vi "stdin.write.vi"(8 "error in (no error)":errorcluster, 10 "stdin":string, 11 "dotnet_system_exec in":refnum<class "dotnet_system_exec.lvclass">) -> (0 "error out":errorcluster, 3 "dotnet_system_exec out":refnum<class "dotnet_system_exec.lvclass">)   [LabVIEW 2015, in "dotnet_system_exec.lvclass"]
doc: "Sends a line to the .NET process via stdin. This vi accepts multiline inputs in case multiple lines want to be sent at once."
uses:
  dotnet_system_exec.lvclass
  dotnet_system_exec.lvclass/dotnet_system_exec.ctl
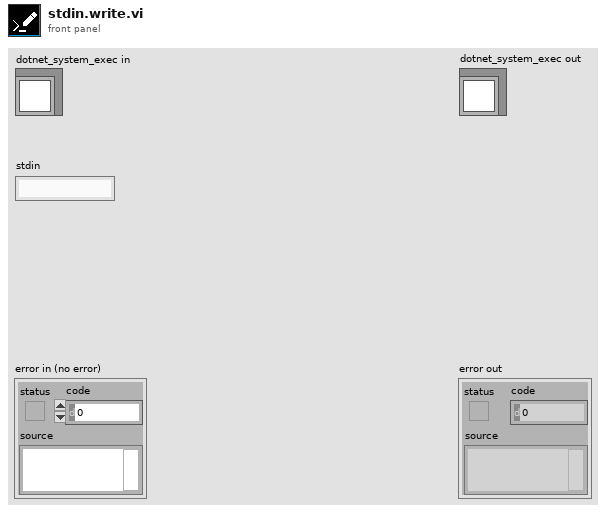
[diagram p1: front panel]
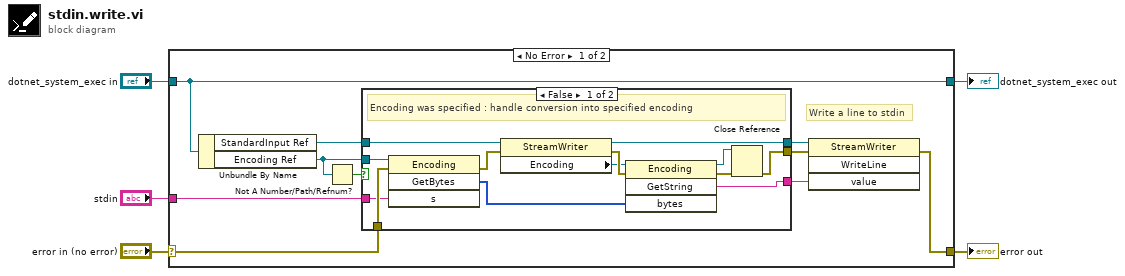
[diagram p0: block diagram]
diagram:
  n1 = case shown="No Error" "error in (no error)" {
    selector: "error in (no error)" -> [w9 w33]
    tunnel: [w13 w33] -> w4
    tunnel: [w15 w32] -> w2
    tunnel: "dotnet_system_exec in" -> [w15 w32]
    tunnel: "stdin" -> [w10 _]
    frame No Error {
      # "Write a line to stdin"
      n2 = Unbundle By Name(w15) -> ("StandardInput Ref"=w14:refnum<k24>, "Encoding Ref"=w7:refnum<k24>)
      n3 = Not A Number/Path/Refnum?(number/path/refnum=w7) -> (NaN/Path/Refnum?=w8:bool)
      n4 = case shown="False" w8 {
        tunnel: w14 -> [w26 w31]
        tunnel: [w25 w31] -> w12
        tunnel: [w23 w30] -> w11
        tunnel: w10 -> [w22 w30]
        tunnel: w7 -> [w20 _]
        tunnel: w9 -> [w27 w29]
        tunnel: [w16 w29] -> w6
        frame False {
          # "Encoding was specified : handle conversion into specified encoding"
          n5 = invoke class="Encoding" method="GetBytes"(reference=w20, error in=w27, "s"=w22) -> (error out=w19:errorcluster, "GetBytes"=w24:u8[])  [unwired: 1 in, 2 out]
          n6 = property class="StreamWriter"(reference=w26, error in=w19) -> (reference out=w25:refnum<k24>, error out=w28:errorcluster, "Encoding"=w21:refnum<k24>)
          n7 = invoke class="Encoding" method="GetString"(reference=w21, error in=w28, "bytes"=w24) -> (reference out=w17:refnum<k24>, error out=w18:errorcluster, "GetString"=w23:string)  [unwired: 1 in, 1 out]
          n8 = Close Reference(reference=w17, error in (no error)=w18) -> (error out=w16:errorcluster)
        }
        frame True {
        }
      }
      n9 = invoke class="StreamWriter" method="WriteLine"(reference=w12, error in=w6, "value"=w11) -> (error out=w13:errorcluster)  [unwired: 1 in, 3 out]
    }
    frame Error {
    }
  }
  "error out" <- w4
  "dotnet_system_exec out" <- w2
